vi "Differentiation.vi"(5 "formula":string, 6 "end":dbl=1.0 format="%.2f", 7 "start":dbl format="%.2f", 8 "number of points":u32=10) -> (0 "ticks":u32, 1 "error":i32, 2 "Derivative of Y":dbl[](array[numeric]) format="%.2f", 3 "Y Values":dbl[](array[numeric]) format="%.2f", 4 "X Values":dbl[](array[numeric]) format="%.2f")   [LabVIEW 2017, in "NI_Gmath.lvlib"]
doc: "Calculates both function values and the values of the derivative of a given 1D function defined by a formula at equidistant points in an interval."
uses:
  <vilib>/gmath/NI_Gmath.lvlib
panel:
  # "Example:\n\n number of points: 100 \n start: 0.0\n end: 1.0\n formula: sin(t)+cos(t)"
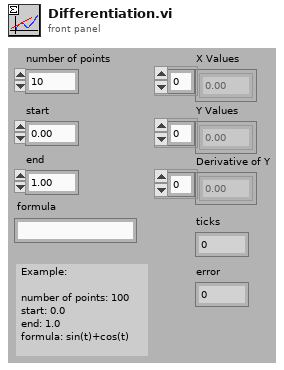
[diagram p1: front panel]
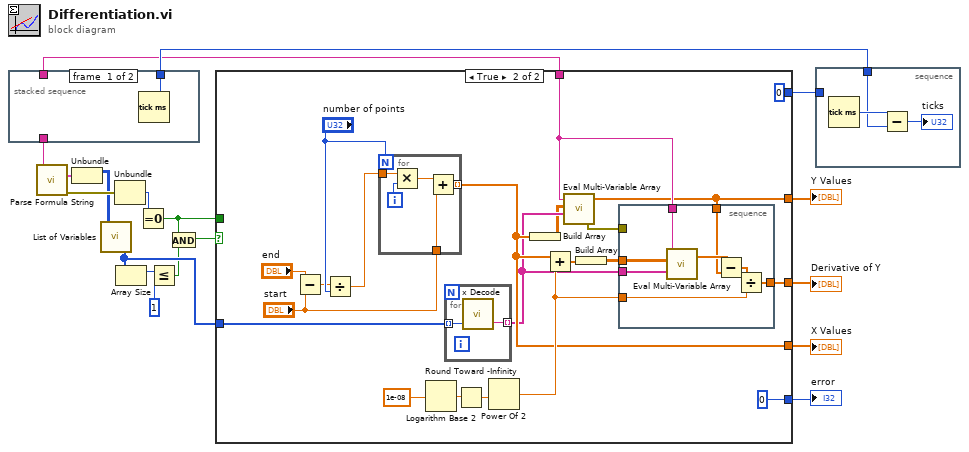
[diagram p0: block diagram]
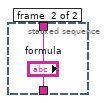
[diagram p2: hidden frame]
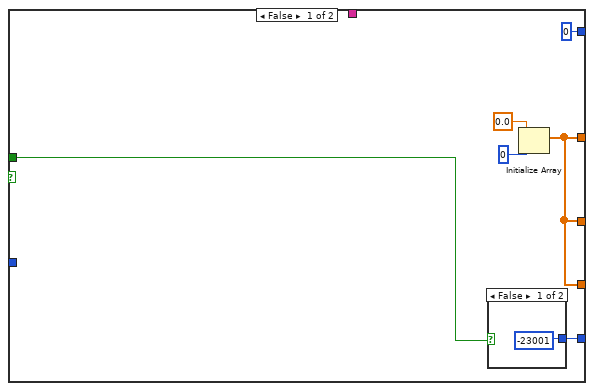
[diagram p3: hidden frame]
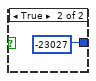
[diagram p4: hidden frame]
diagram:
  n1 = stacked-sequence {
    tunnel: [w19 _] -> w14
    tunnel: [_ "formula"] -> w2
    tunnel: [_ "formula"] -> w1
    frame #0 {
      n2 = Tick Count (ms)() -> (millisecond timer value=w19:u32)
    }
    frame #1 {
    }
  }
  n3 = call <vilib>:"Parse Formula String.vi"("formula"=w1) -> ("error out"=w9:errorcluster, "Parsed Formula"=w4:cluster{"Table":i32[][], "Y Values":dbl[]})  [unwired: 1 in]
  n4 = Unbundle(w4) -> ("Table"=w3:i32[][])  [unwired: 1 out]
  n5 = call <vilib>:"List of Variables.vi"("Table"=w3) -> ("List of variables"=w15:i32[])
  n6 = Unbundle(w9) -> ("code"=w8:i32)  [unwired: 2 out]
  n7 = Array Size(array=w15) -> (size(s)=w17:i32)
  n8 = Equal To 0?(x=w8) -> (x = 0?=w5:bool)
  n9 = Less Or Equal?(x=w17, y=1) -> (x <= y?=w6:bool)
  n10 = And(x=w5, y=w6) -> (x .and. y?=w18:bool)
  n11 = case shown="True" w18 {
    tunnel: w2 -> [_ w49]
    tunnel: w15 -> [_ w48]
    tunnel: [w23 w35] -> w13
    tunnel: [w23 w34] -> w12
    tunnel: [w23 w33] -> w11
    tunnel: [0 0] -> w10
    tunnel: [w22 0] -> w7
    tunnel: w5 -> [w21 _]
    frame False {
      n12 = case shown="False" w21 {
        tunnel: [-23001 -23027] -> w22
        frame False {
        }
        frame True {
        }
      }
      n13 = Initialize Array(0.0, 0) -> (w23:dbl[])
    }
    frame True {
      n14 = Subtract(x="end", y="start") -> (x-y=w36:dbl)
      n15 = Divide(x=w36, y="number of points") -> (x/y=w37:dbl)
      n16 = for {
        N: "number of points" -> [_]
        tunnel: w37 -> [w54]
        tunnel: "start" -> [w51]
        tunnel: [w50] -> w33 mode=indexing
        i -> [w53]
        n17 = Multiply(x=w54, y=w53) -> (x*y=w52:dbl)
        n18 = Add(x=w52, y=w51) -> (x+y=w50:dbl)
      }
      n19 = Logarithm Base 2(1:1e-08) -> (0:w44:dbl)
      n20 = for {
        tunnel: w48 -> [w56] mode=indexing
        tunnel: [w55] -> w31 mode=indexing
        n21 = call <vilib>:"x Decode.vi"("number"=w56) -> ("x string"=w55:string)  [unwired: 1 in, 1 out]
      }
      n22 = Round Toward -Infinity(1:w44) -> (0:w45:dbl)
      n23 = Power Of 2(x=w45) -> (2^x=w46:dbl)
      n24 = Build Array(w33) -> (w30:dbl[][])
      n25 = Add(x=w33, y=w46) -> (x+y=w42:dbl[])
      n26 = call <vilib>:"Eval Multi-Variable Array.vi"("Variables"=w31, "X Values"=w30, "formula"=w49) -> ("error out"=w39:errorcluster, "Y Values"=w35:dbl[])  [unwired: 1 in]
      n27 = Build Array(w42) -> (w43:dbl[][])
      n28 = stacked-sequence {
        tunnel: w39 -> [_]
        tunnel: w49 -> [w64]
        tunnel: w31 -> [w57]
        tunnel: w43 -> [w58]
        tunnel: w35 -> [w62]
        tunnel: w46 -> [w60]
        tunnel: [w59] -> w34
        frame #0 {
          n29 = call <vilib>:"Eval Multi-Variable Array.vi"("Variables"=w57, "X Values"=w58, "formula"=w64) -> ("Y Values"=w63:dbl[])  [unwired: 1 in, 1 out]
          n30 = Subtract(x=w63, y=w62) -> (x-y=w61:dbl[])
          n31 = Divide(x=w61, y=w60) -> (x/y=w59:dbl[])
        }
      }
    }
  }
  "error" <- w7
  "X Values" <- w11
  "Y Values" <- w13
  "Derivative of Y" <- w12
  n32 = stacked-sequence {
    tunnel: w14 -> [w65]
    tunnel: w10 -> [_]
    frame #0 {
      n33 = Tick Count (ms)() -> (millisecond timer value=w66:u32)
      n34 = Subtract(x=w66, y=w65) -> (x-y=→"ticks":u32)
    }
  }
